vi "Get Named Ranges.vi"(8 "error in":errorcluster, 10 "Sheet Name":string, 11 "SpreadsheetDoc in":refnum<k24>) -> (0 "error out":errorcluster, 1 "Cells":cluster{"Cells":variant[][]}[](array[cluster]), 2 "Range Names":string[](array[string]), 3 "SpreadsheetDoc out":refnum<k24>)   [LabVIEW 2019, in "Open Xml.lvlib"]
uses:
  Open Xml.lvlib
  D:/git/Open-Xml-LabVIEW/Source/DocumentFormat.OpenXml.dll
  DocumentFormat.OpenXml.dll
  D:/git/Open-Xml-LabVIEW/Source/DocumentFormat.OpenXml.Framework.dll
  DocumentFormat.OpenXml.Framework.dll
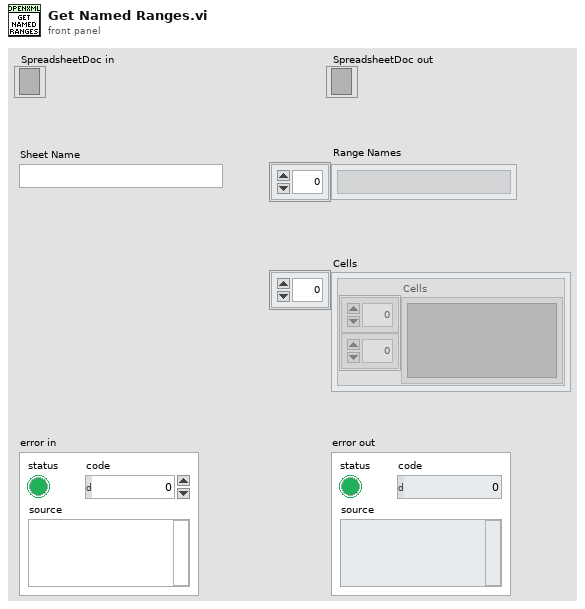
[diagram p1: front panel]
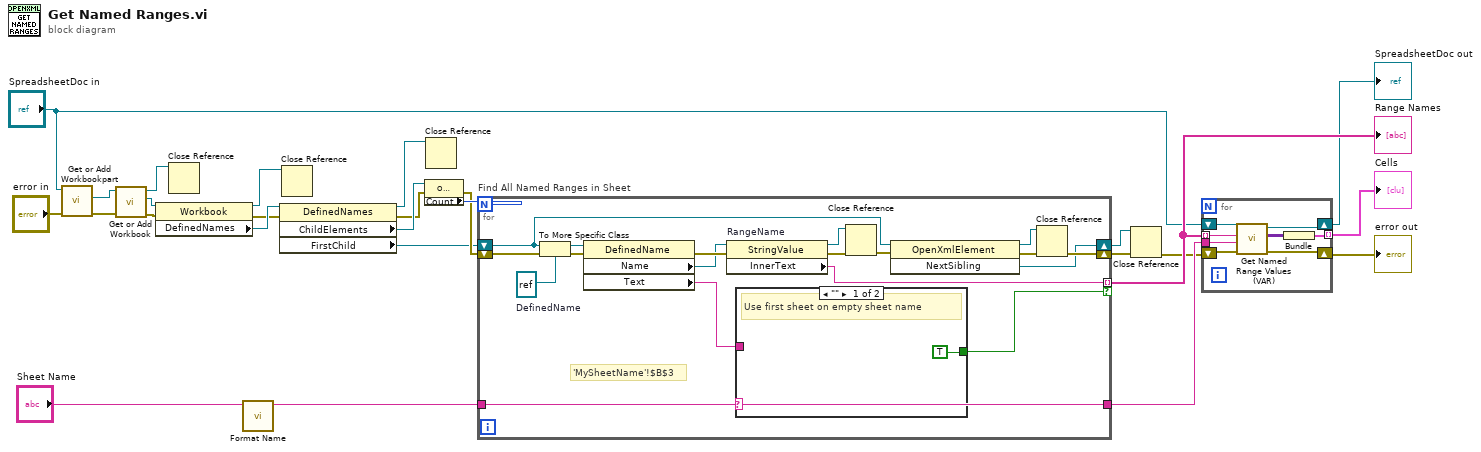
[diagram p0: block diagram]
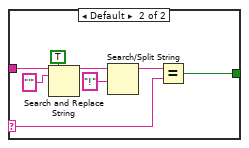
[diagram p2: hidden frame]
diagram:
  n1 = call "Get or Add Workbookpart.vi"("error in"="error in", "SpreadsheetDoc in"="SpreadsheetDoc in") -> ("error out"=w13:errorcluster, "WorkbookPart"=w10:refnum<k24>)  [unwired: 7 in, 1 out]
  n2 = call "Get or Add Workbook.vi"("error in"=w13, "Workbookpart in"=w10) -> ("error out"=w14:errorcluster, "Workbook"=w11:refnum<k24>, "Workbookpart out"=w3:refnum<k24>)  [unwired: 7 in]
  n3 = property class="Workbook"(reference=w11, error in=w14) -> (reference out=w25:refnum<k24>, error out=w12:errorcluster, "DefinedNames"=w26:refnum<k24>)
  n4 = Close Reference(reference=w3) -> ()  [unwired: 1 in, 1 out]
  n5 = call "Format Name.vi"("Sheet Name"="Sheet Name") -> ("Formatted Sheet Name"=w1:string)  [unwired: 10 in]
  n6 = property class="DefinedNames"(reference=w26, error in=w12) -> (reference out=w24:refnum<k24>, error out=w7:errorcluster, "ChildElements"=w9:refnum<k24>, "FirstChild"=w4:refnum<k24>)
  n7 = Close Reference(reference=w25) -> ()  [unwired: 1 in, 1 out]
  n8 = property class="OpenXmlElementList"(reference=w9, error in=w7) -> (error out=w6:errorcluster, "Count"=w8:i32)  [unwired: 1 out]
  n9 = Close Reference(reference=w24) -> ()  [unwired: 1 in, 1 out]
  n10 = for "Find All Named Ranges in Sheet" {
    N: w8 -> [_]
    shift-right: [w42] -> w21
    shift-left: w6 -> [w33]
    tunnel: w1 -> [w34]
    shift-right: [w40] -> w17
    shift-left: w4 -> [w27]
    tunnel: [w36] -> w22 mode=indexing if=w35
    tunnel: [w34] -> w19
    w41 = refnum<k24> refnum  # DefinedName
    # "'MySheetName'!$B$3"
    n11 = To More Specific Class(target class=w41, reference=w27, error in=w33) -> (specific class reference=w44:refnum<k24>, error out=w43:errorcluster)
    n12 = property class="DefinedName"(reference=w44, error in=w43) -> (error out=w32:errorcluster, "Name"=w30:refnum<k24>, "Text"=w31:string)  [unwired: 1 out]
    n13 = property on="RangeName" class="StringValue"(reference=w30, error in=w32) -> (reference out=w39:refnum<k24>, error out=w29:errorcluster, "InnerText"=w36:string)
    n14 = case shown="\"\"" w34 {
      selector: w34 -> [_ w48]
      tunnel: [TRUE w49] -> w35
      tunnel: w31 -> [_ w46]
      frame "" {
        # "Use first sheet on empty sheet name"
      }
      frame Default {
        n15 = Search and Replace String(replace all?=TRUE ("replace all? (F)"), input string=w46, search string="'") -> (result string=w53:string)  [unwired: 5 in, 3 out]
        n16 = Search/Split String(string=w53, search string/char (-)="!") -> (substring before match=w47:string)  [unwired: 1 in, 2 out]
        n17 = Equal?(x=w47, y=w48) -> (x = y?=w49:bool)
      }
    }
    n18 = Close Reference(reference=w39, error in (no error)=w29) -> (error out=w28:errorcluster)
    n19 = invoke class="OpenXmlElement" method="NextSibling"(reference=w27, error in=w28) -> (reference out=w37:refnum<k24>, error out=w38:errorcluster, "NextSibling"=w40:refnum<k24>)  [unwired: 1 in]
    n20 = Close Reference(reference=w37, error in (no error)=w38) -> (error out=w42:errorcluster)
  }
  "Range Names" <- w22
  n21 = Close Reference(reference=w17, error in (no error)=w21) -> (error out=w18:errorcluster)
  n22 = for {
    tunnel: w22 -> [w61] mode=indexing
    shift-right: [w58] -> w20
    shift-left: w18 -> [w60]
    tunnel: w19 -> [w59]
    shift-right: [w55] -> w5
    shift-left: "SpreadsheetDoc in" -> [w54]
    tunnel: [w56] -> w16 mode=indexing
    n23 = call "Get Named Range Values (VAR).vi"("error in"=w60, "Sheet Name"=w59, "Named Range Identifier"=w61, "SpreadsheetDoc in"=w54) -> ("error out"=w58:errorcluster, "Cells"=w57:variant[][], "SpreadsheetDoc out"=w55:refnum<k24>)  [unwired: 5 in]
    n24 = Bundle("Cells"=w57) -> (w56:cluster{"Cells":variant[][]})  [unwired: 1 in]
  }
  "SpreadsheetDoc out" <- w5
  "error out" <- w20
  "Cells" <- w16
